vi "Write Controls to Config File.vi"(8 "error in (no error)":errorcluster, 10 "Control References":refnum<vi>[](array[refnum]), 11 "Configuration File Reference In":T1) -> (0 "error out":errorcluster, 3 "Configuration File Reference Out":T1)   [LabVIEW 2020]
doc: "Writes the values of an array of controls to a configuration file.\nControl References is an array of the references of the controls to be saved.\n\nThe section name is the name of the VI that holds the control.\nThe key name is the label of the control."
uses:
  <vilib>/Utility/config.llb/Config Data RefNum.ctl
  <vilib>/Utility/config.llb/NI_LVConfig.lvlib
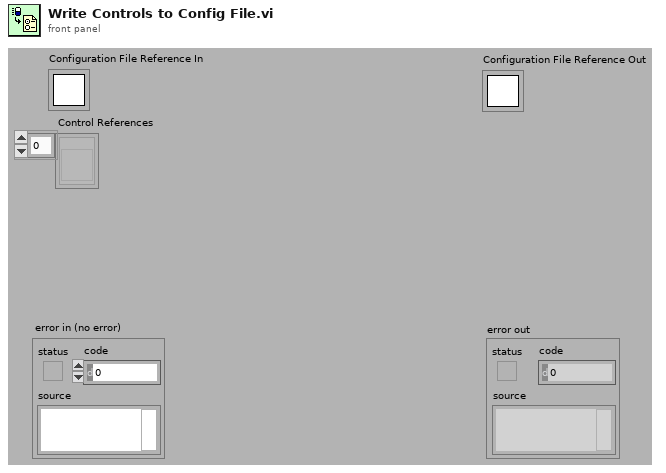
[diagram p1: front panel]
types:
  T1 = typedef "NI_LVConfig.lvlib/Config Data RefNum.ctl" = refnum<k1>
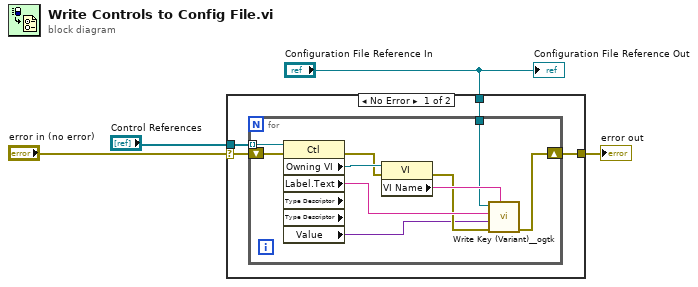
[diagram p0: block diagram]
diagram:
  n1 = case shown="No Error" "error in (no error)" {
    selector: "error in (no error)" -> [w5 w19]
    tunnel: "Control References" -> [w8 _]
    tunnel: [w7 w19] -> w3
    tunnel: "Configuration File Reference In" -> [w6 _]
    frame No Error {
      n2 = for {
        tunnel: w8 -> [w18] mode=indexing
        shift-right: [w11] -> w7
        shift-left: w5 -> [w12]
        tunnel: w6 -> [w10]
        n3 = property class="Ctl" props=["Owning VI", "Label", "Text", "Type Descriptor", "Type Descriptor", "Value"](reference=w18, error in=w12) -> (error out=w14:errorcluster, "Owning VI"=w17:refnum<vi>, "Label.Text"=w15:string, "Value"=w9:variant)  [unwired: 3 out]
        n4 = property class="VI"(reference=w17, error in=w14) -> (error out=w13:errorcluster, "VI Name"=w16:string)  [unwired: 1 out]
        n5 = call <userlib>:"Write Key (Variant)__ogtk.vi"("section"=w16, "error in (no error)"=w13, "key-value"=w9, "key (optional)"=w15, "refnum"=w10) -> ("error out"=w11:errorcluster)  [unwired: 5 in, 1 out]
      }
    }
    frame Error {
    }
  }
  "error out" <- w3
  "Configuration File Reference Out" <- "Configuration File Reference In"
